vi "Sort.vi"   [LabVIEW 2018]
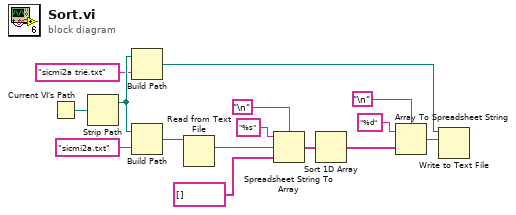
[diagram p0: block diagram]
diagram:
  n1 = Current VI's Path() -> (path=w14:path)
  n2 = Strip Path(path=w14) -> (stripped path=w3:path)  [unwired: 1 out]
  n3 = Build Path(base path=w3, name or relative path="sicmi2a trié.txt") -> (appended path=w1:path)
  n4 = Build Path(base path=w3, name or relative path="sicmi2a.txt") -> (appended path=w13:path)
  n5 = Read from Text File(file (use dialog)=w13) -> (text=w11:string)  [unwired: 3 in, 3 out]
  n6 = Spreadsheet String To Array(delimiter (Tab)="\n", format string="%s", spreadsheet string=w11, array type (2D Dbl)=string[] []) -> (array=w8:string[])
  n7 = Sort 1D Array(array=w8) -> (sorted array=w7:string[])
  n8 = Array To Spreadsheet String(delimiter (Tab)="\n", array=w7, 3:"%d" ("format string")) -> (spreadsheet string=w4:string)
  n9 = Write to Text File(file (use dialog)=w1, text=w4) -> ()  [unwired: 2 in, 3 out]
